vi "Write Step Configuration.vi"(8 "error in (no error)":errorcluster, 10 "Measurement Actor.lvlib:Step Configuration.lvclass":refnum<class "Step Configuration.lvclass">, 11 "Measurement Data in":refnum<class "Measurement Data.lvclass">) -> (0 "error out":errorcluster, 3 "Measurement Data out":refnum<class "Measurement Data.lvclass">)   [LabVIEW 2016, in "Measurement Setup Controller.lvlib" / "Measurement Data.lvclass"]
uses:
  Measurement Data.lvclass
  MAL-Framework/user.lib/Common Components/Measurement Actor/Configuration/Step Configuration.lvclass
  Measurement Data.lvclass/Measurement Data.ctl
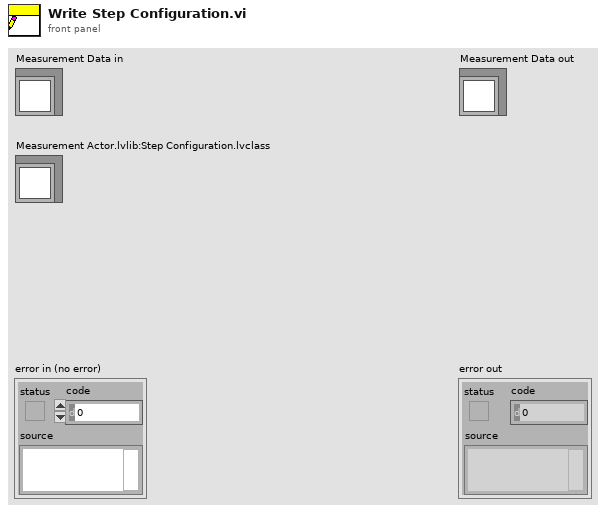
[diagram p1: front panel]
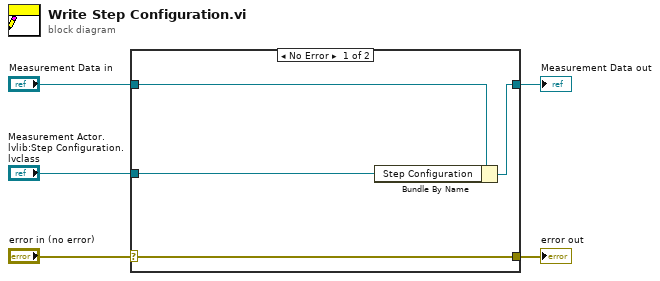
[diagram p0: block diagram]
diagram:
  n1 = case shown="No Error" "error in (no error)" {
    selector: "error in (no error)" -> [w9 w10]
    tunnel: [w9 w10] -> w4
    tunnel: [w7 w11] -> w2
    tunnel: "Measurement Data in" -> [w8 w11]
    tunnel: "Measurement Actor.lvlib:Step Configuration.lvclass" -> [w6 _]
    frame No Error {
      n2 = Bundle By Name(cluster=w8, "Step Configuration"=w6) -> (w7:refnum<class "Measurement Data.lvclass">)
    }
    frame Error {
    }
  }
  "error out" <- w4
  "Measurement Data out" <- w2
